vi "ObjectIntoKeeperArea.vi"(8 "error in (no error)":errorcluster, 9 "ObjectAttackerPosition(FA)":dbl[](array[numeric]), 10 "FieldRef":refnum<class "Field.lvclass">, 11 "Utilities in":refnum<class "Utilities.lvclass">) -> (0 "error out":errorcluster, 1 "IntoTheirsArea?":bool=TRUE, 2 "IntoOursArea?":bool=TRUE, 3 "Utilities out":refnum<class "Utilities.lvclass">)   [LabVIEW 2023, in "Utilities.lvclass"]
uses:
  Utilities.lvclass
  Field_class/Field.lvclass
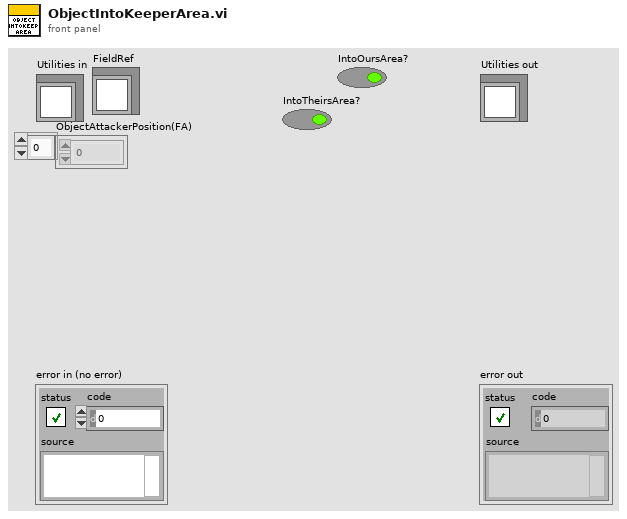
[diagram p1: front panel]
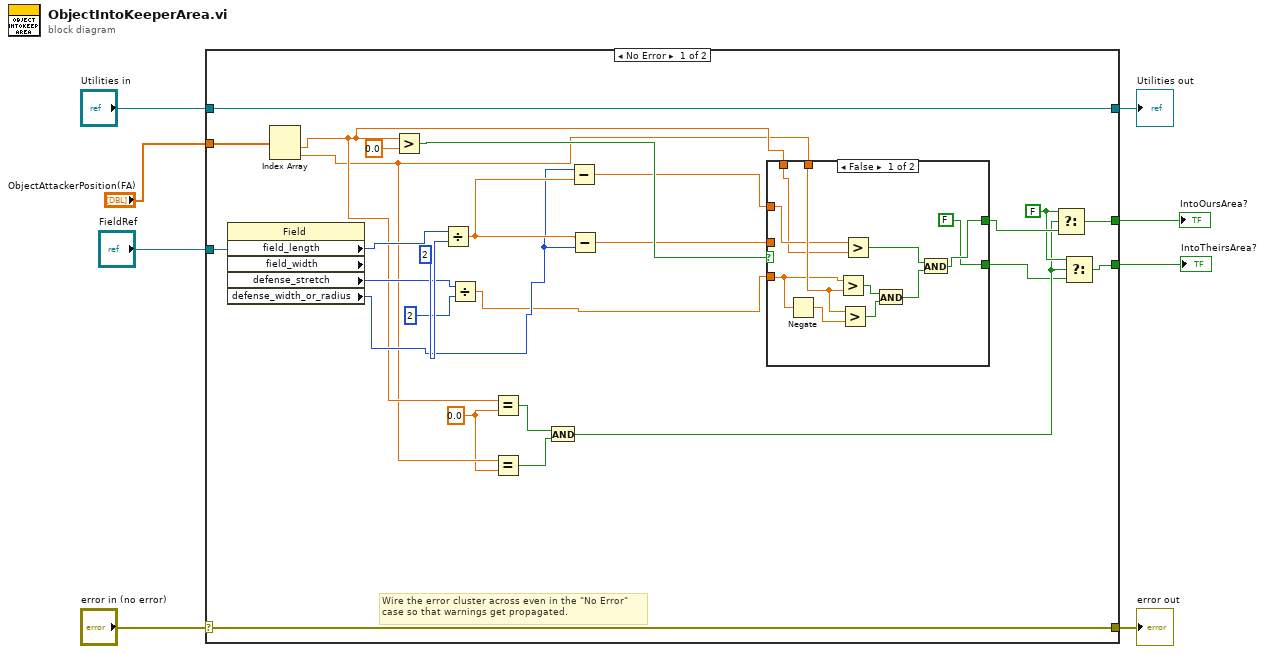
[diagram p0: block diagram]
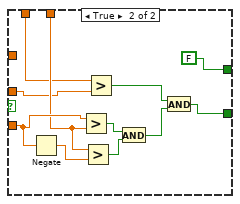
[diagram p2: hidden frame]
diagram:
  n1 = case shown="No Error" "error in (no error)" {
    selector: "error in (no error)" -> [w33 w58]
    tunnel: [w33 w58] -> w7
    tunnel: [w34 w57] -> w5
    tunnel: "Utilities in" -> [w34 w57]
    tunnel: "FieldRef" -> [w32 _]
    tunnel: "ObjectAttackerPosition(FA)" -> [w29 _]
    tunnel: [w9 _] -> w2
    tunnel: [w13 _] -> w1
    frame No Error {
      w12 = FALSE ("t")
      w17 = 0.0 ("y")
      # "Wire the error cluster across even in the \"No Error\"\ncase so that warnings get propagated."
      n2 = property class="Field" props=["field_length", "field_width", "defense_stretch", "defense_width_or_radius"](reference=w32) -> ("field_length"=w31:i32, "defense_stretch"=w22:i32, "defense_width_or_radius"=w21:i32)  [unwired: 1 in, 3 out]
      n3 = Index Array(array=w29) -> (element #1=w19:dbl, element #2=w18:dbl)  [unwired: 2 in]
      n4 = Greater?(x=w19, y=0.0) -> (0:w27:bool)
      n5 = Divide(x=w31, y=2) -> (x/y=w26:dbl)
      n6 = Divide(x=w22, y=2) -> (x/y=w20:dbl)
      n7 = Equal?(x=w19, y=w17) -> (x = y?=w16:bool)
      n8 = Equal?(x=w18, y=w17) -> (x = y?=w15:bool)
      n9 = And(x=w16, y=w15) -> (x .and. y?=w11:bool)
      n10 = Subtract(x=w21, y=w26) -> (x-y=w24:dbl)
      n11 = Subtract(x=w26, y=w21) -> (x-y=w25:dbl)
      n12 = case shown="False" w27 {
        tunnel: w25 -> [_ w47]
        tunnel: w18 -> [w40 w55]
        tunnel: w19 -> [w38 w46]
        tunnel: w20 -> [w37 w56]
        tunnel: [FALSE w49] -> w10
        tunnel: [w36 FALSE] -> w14
        tunnel: w24 -> [w39 _]
        frame False {
          n13 = Negate(x=w37) -> (-x=w45:dbl)
          n14 = Greater?(x=w37, y=w40) -> (0:w44:bool)
          n15 = Greater?(x=w40, y=w45) -> (0:w43:bool)
          n16 = Greater?(x=w39, y=w38) -> (0:w41:bool)
          n17 = And(x=w44, y=w43) -> (x .and. y?=w42:bool)
          n18 = And(x=w41, y=w42) -> (x .and. y?=w36:bool)
        }
        frame True {
          n19 = Negate(x=w56) -> (-x=w54:dbl)
          n20 = Greater?(x=w56, y=w55) -> (0:w53:bool)
          n21 = Greater?(x=w55, y=w54) -> (0:w52:bool)
          n22 = Greater?(x=w46, y=w47) -> (0:w50:bool)
          n23 = And(x=w53, y=w52) -> (x .and. y?=w51:bool)
          n24 = And(x=w50, y=w51) -> (x .and. y?=w49:bool)
        }
      }
      n25 = Select(t=w12, s=w11, f=w14) -> (s? t:f=w13:bool)
      n26 = Select(t=w12, s=w11, f=w10) -> (s? t:f=w9:bool)
    }
    frame Error {
    }
  }
  "error out" <- w7
  "Utilities out" <- w5
  "IntoOursArea?" <- w1
  "IntoTheirsArea?" <- w2
